vi "Barcode(SN)Single.vi"(6 "Model":string, 7 "Station":string, 8 "Button-OK":bool, 10 "menu reference":refnum<k9>, 11 "Barcode(S/N):":string) -> (0 "Stop":bool=TRUE, 2 "SNCheck":bool, 3 "Barcode out:":string, 4 "Model":string)   [LabVIEW 2013]
uses:
  <vilib>/event_ctls.llb/eventvkey.ctl
panel:
  in  "Button-Cancel":bool
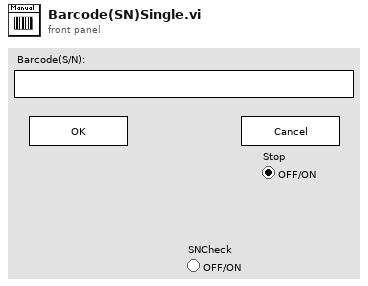
[diagram p1: front panel]
types:
  T1 = typedef "eventvkey.ctl" = enum16{"ASCII", "Enter", "Return", "Shift", "Ctrl", "Alt", "Cmd", "Opt", "Caps", "NumLock", "Clear", "Break", "Up", "Down", "Left", "Right", "Insert", "Delete", "Home", "End", "PageUp", "PageDown", "Escape", "Help", "Pause", "ScrollLock", "F1", "F2", "F3", "F4", "F5", "F6", "F7", "F8", "F9", "F10", "F11", "F12", "F13", "F14", "F15", "F16", "F17", "F18", "F19", "F20", "F21", "F22", "F23", "F24", "Play", "VolumeUp", "VolumeDown", "Mute", "Two Byte Char"}
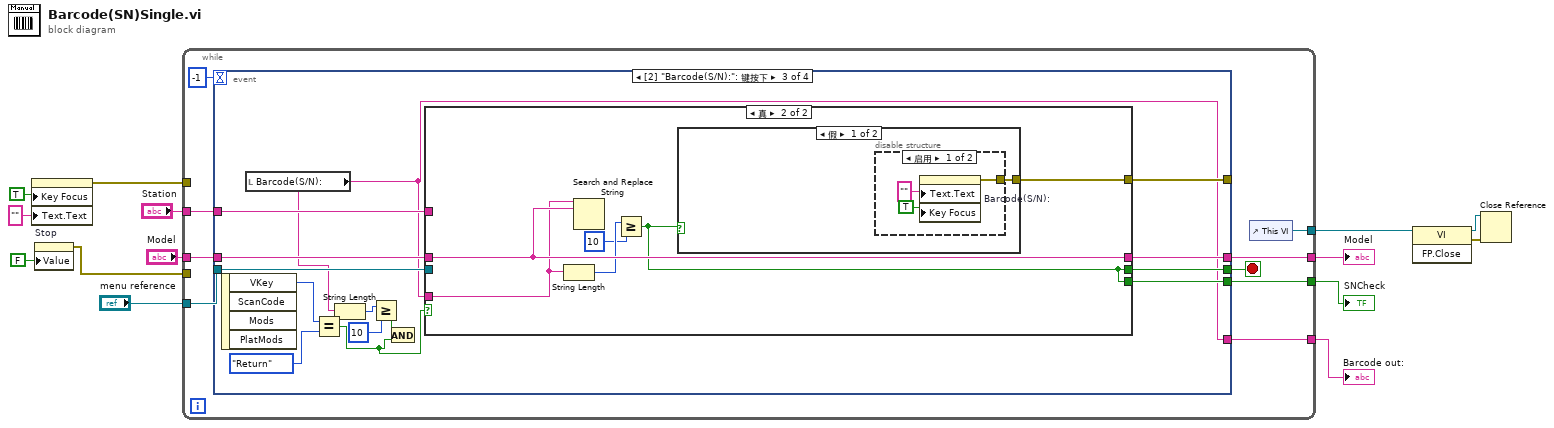
[diagram p0: block diagram]
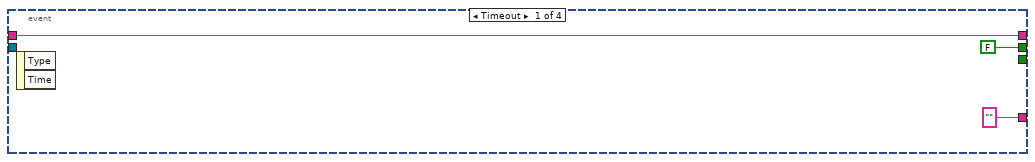
[diagram p2: hidden frame]
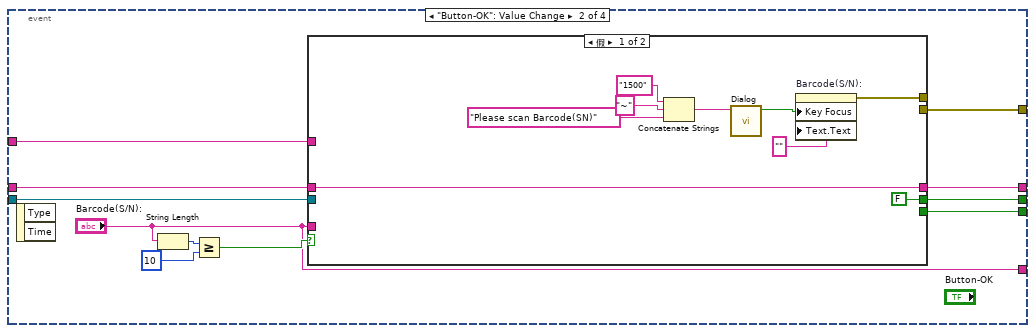
[diagram p3: hidden frame]
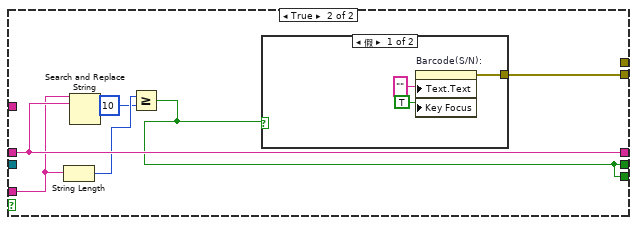
[diagram p4: hidden frame]
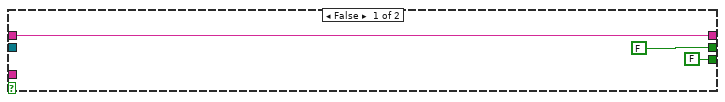
[diagram p6: hidden frame]
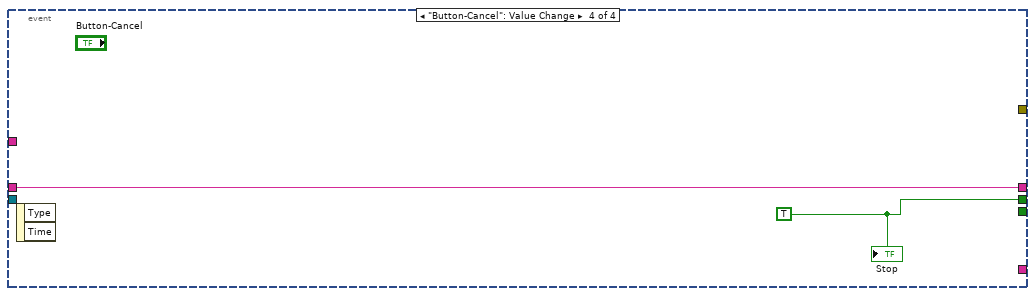
[diagram p9: hidden frame]
diagram:
  n1 = property on="Barcode(S/N):" class="Str"("Key Focus"=TRUE, "Text.Text"="" ("文本.文本")) -> (error out=w9:errorcluster)  [unwired: 2 in, 1 out]
  n2 = property on="Stop" class="Bool (严格)"("Value"=FALSE ("Stop")) -> (error out=w3:errorcluster)  [unwired: 2 in, 1 out]
  n3 = while {
    tunnel: [w23] -> w11
    tunnel: [w22] -> w10
    tunnel: w9 -> [_]
    tunnel: "Model" -> [w20]
    tunnel: [w19] -> w8
    tunnel: "Station" -> [w18]
    tunnel: "menu reference" -> [w17]
    tunnel: [w16] -> w4
    tunnel: w3 -> [_]
    stop <- w21 stop-if-true
    n4 = event shown="[2] \"Barcode(S/N):\": 键按下" {
      selector: _ -> [_ _ _ _]
      dyn-events: _ -> [_ _ _ _]
      timeout: -1 -> [_ _ _ _]
      tunnel: [FALSE ("OK in") w36 w69 w84] -> w21
      tunnel: ["" ("Barcode:") "Barcode(S/N):" w62 _] -> w22
      tunnel: [_ w34 w68 _] -> _
      tunnel: w20 -> [w24 w33 w67 w83]
      tunnel: [w24 w32 w66 w83] -> w19
      tunnel: w18 -> [_ w31 w65 _]
      tunnel: w17 -> [_ w30 w64 _]
      tunnel: [_ w29 w63 _] -> w16
      event Timeout {
        n5 = event-data() -> ()  [unwired: 1 in, 2 out]
      }
      event "Button-OK": Value Change {
        n6 = event-data() -> ()  [unwired: 1 in, 2 out]
        n7 = String Length(string="Barcode(S/N):") -> (length=w28:i32)
        n8 = Greater Or Equal?(x=w28, y=10) -> (x >= y?=w37:bool)
        n9 = case shown="假" w37 {
          tunnel: [FALSE ("OK in") w47] -> w36
          tunnel: [w45 _] -> _
          tunnel: "Barcode(S/N):" -> [_ w50]
          tunnel: [_ w52] -> w34
          tunnel: w33 -> [w39 w51]
          tunnel: [w39 w51] -> w32
          tunnel: w31 -> [_ _]
          tunnel: w30 -> [_ _]
          tunnel: [_ w47] -> w29
          frame False {
            n10 = Concatenate Strings("1500" ("string"), "~" ("string"), "Please scan Barcode(SN)" ("message")) -> (w41:string)
            n11 = call "Dialog.vi"("Limit"=w41) -> ("true"=w40:bool)  [unwired: 9 in, 1 out]
            n12 = property on="Barcode(S/N):" class="Str"("Key Focus"=w40, "Text.Text"="" ("文本.文本")) -> (error out=w45:errorcluster)  [unwired: 2 in, 1 out]
          }
          frame True {
            n13 = String Length(string=w50) -> (length=w49:i32)
            n14 = Search and Replace String(input string=w50, search string=w51) -> ()  [unwired: 6 in, 4 out]
            n15 = Greater Or Equal?(x=w49, y=10) -> (x >= y?=w47:bool)
            n16 = case shown="假" w47 {
              tunnel: [w54 _] -> w52
              frame False {
                n17 = property on="Barcode(S/N):" class="Str"("Text.Text"="", "Key Focus"=TRUE) -> (error out=w54:errorcluster)  [unwired: 2 in, 1 out]
              }
              frame True {
              }
            }
          }
        }
      }
      event "Barcode(S/N):": Key Down {
        n18 = event-data() -> ("VKey"=w61:T1)  [unwired: 1 in, 3 out]
        n19 = local read "Barcode(S/N):"() -> (w62:string)
        n20 = Equal?(x=w61, y=eventvkey."Return" ("VKey")) -> (x = y?=w56:bool)
        n21 = String Length(string=w62) -> (length=w59:i32)
        n22 = Greater Or Equal?(x=w59, y=10) -> (x >= y?=w57:bool)
        n23 = And(x=w57, y=w56) -> ()  [unwired: 1 out]
        n24 = case shown="真" w56 {
          tunnel: [FALSE ("OK in") w76] -> w69
          tunnel: w62 -> [_ w75]
          tunnel: [_ w78] -> w68
          tunnel: w67 -> [w71 w77]
          tunnel: [w71 w77] -> w66
          tunnel: w65 -> [_ _]
          tunnel: w64 -> [_ _]
          tunnel: [FALSE w76] -> w63
          frame False {
          }
          frame True {
            n25 = String Length(string=w75) -> (length=w74:i32)
            n26 = Search and Replace String(input string=w75, search string=w77) -> ()  [unwired: 6 in, 4 out]
            n27 = Greater Or Equal?(x=w74, y=10) -> (x >= y?=w76:bool)
            n28 = case shown="假" w76 {
              tunnel: [w79 _] -> w78
              frame False {
                n29 = disable-structure shown="启用" {
                  disable-tunnel: [w81 _] -> w79
                  frame Enabled {
                    n30 = property on="Barcode(S/N):" class="Str"("Text.Text"="", "Key Focus"=TRUE) -> (error out=w81:errorcluster)  [unwired: 2 in, 1 out]
                  }
                  frame Disabled {
                  }
                }
              }
              frame True {
              }
            }
          }
        }
      }
      event "Button-Cancel": Value Change {
        w84 = TRUE ("OK in")
        n31 = event-data() -> ()  [unwired: 1 in, 2 out]
        "Stop" <- w84
      }
    }
    n32 = control-ref of="This VI"() -> (w23:refnum<vi>)
  }
  "Barcode out:" <- w10
  "Model" <- w8
  "SNCheck" <- w4
  n33 = invoke class="VI" method="FP.Close"(reference=w11) -> (reference out=w13:refnum<vi>, error out=w12:errorcluster)  [unwired: 2 in, 1 out]
  n34 = Close Reference(reference=w13, error in (no error)=w12) -> ()  [unwired: 1 out]
